vi "Read Bus Configuration.vi"(8 "error in":errorcluster, 11 "Bus in":refnum<class "Bus.lvclass">) -> (0 "error out":errorcluster, 1 "Driver Logic Unit":path, 2 "SPI Engine":path, 3 "Bus out":refnum<class "Bus.lvclass">, 4 "alias":string, 5 "SPI Configuration":T1)   [LabVIEW 2014, in "Bus.lvclass"]
uses:
  Bus.lvclass
  Bus Configuration/SPI Configuration.ctl
  Bus.lvclass/Bus.ctl
  Bus Configuration/Bus Configuration.lvclass/Bus Configuration.ctl
  <vilib>/NI/Configuration Framework/serializable configuration/NISE_CEF_serializable configuration.lvclass
  Bus Configuration/Bus Configuration.lvclass
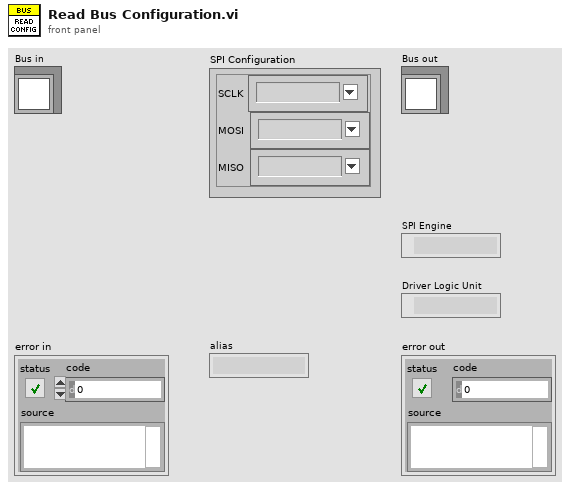
[diagram p1: front panel]
types:
  T1 = typedef "Bus Configuration.lvclass/SPI Configuration.ctl" = cluster{"SCLK":string, "MOSI":string, "MISO":string}
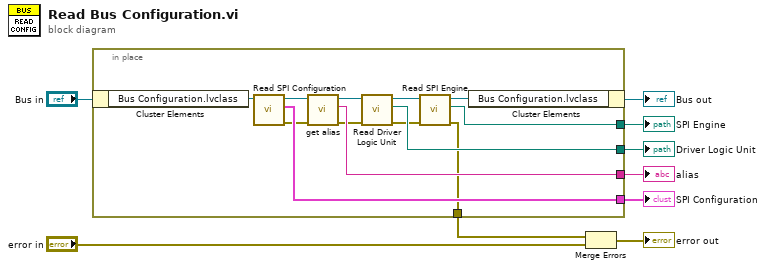
[diagram p0: block diagram]
diagram:
  n1 = in-place {
    in-place-border: [w17] -> w7
    in-place-border: [w16] -> w6
    in-place-border: [w15] -> w5
    in-place-border: [w14] -> w4
    in-place-border: [w10] -> w3
    n2 = in-place-cluster #1("Bus in") -> ("Bus Configuration.lvclass"=w21:refnum<class "Bus Configuration.lvclass">)
    n3 = call "Read SPI Configuration.vi"("Bus Configuration in"=w21) -> ("error out"=w13:errorcluster, "SPI Configuration"=w14:T1, "Bus Configuration out"=w22:refnum<class "Bus Configuration.lvclass">)  [unwired: 8 in]
    n4 = call <vilib>:"get alias.vi"("error in"=w13, "configuration in"=w22) -> ("error out"=w12:errorcluster, "alias"=w15:string, "configuration out"=w20:refnum<class "Bus Configuration.lvclass">)  [unwired: 7 in]
    n5 = call "Read Driver Logic Unit.vi"("error in (no error)"=w12, "Bus Configuration in"=w20) -> ("error out"=w11:errorcluster, "Driver Logic Unit"=w16:path, "Bus Configuration out"=w19:refnum<class "Bus Configuration.lvclass">)  [unwired: 7 in]
    n6 = call "Read SPI Engine.vi"("error in (no error)"=w11, "Bus Configuration in"=w19) -> ("error out"=w10:errorcluster, "SPI Engine"=w17:path, "Bus Configuration out"=w18:refnum<class "Bus Configuration.lvclass">)  [unwired: 7 in]
    n7 = in-place-cluster #1("Bus Configuration.lvclass"=w18) -> (→"Bus out":refnum<class "Bus.lvclass">)
  }
  "SPI Engine" <- w7
  "Driver Logic Unit" <- w6
  "alias" <- w5
  "SPI Configuration" <- w4
  n8 = Merge Errors(w3, "error in") -> (→"error out":errorcluster)
